vi "Is Complete.vi"(8 "error in (no error)":errorcluster, 11 "Measure Controller in":refnum<class "Measure Controller.lvclass">) -> (0 "error out":errorcluster, 3 "Measure Controller out":refnum<class "Measure Controller.lvclass">)   [LabVIEW 2015, in "Measure Controller.lvclass"]
uses:
  Measure Controller.lvclass
  Measure Controller.lvclass/Measure Controller.ctl
  Measure Object/Measure Object.lvclass/Measure Object.ctl
  Measure Object/Read Counter.vi
  Measure Object/Read Repeat times.vi
  Measure Object/Read Reply to.vi
  Measure Object/Write Counter.vi
  Measure Object Messages/Result Reply Msg/Result Reply Msg.lvclass
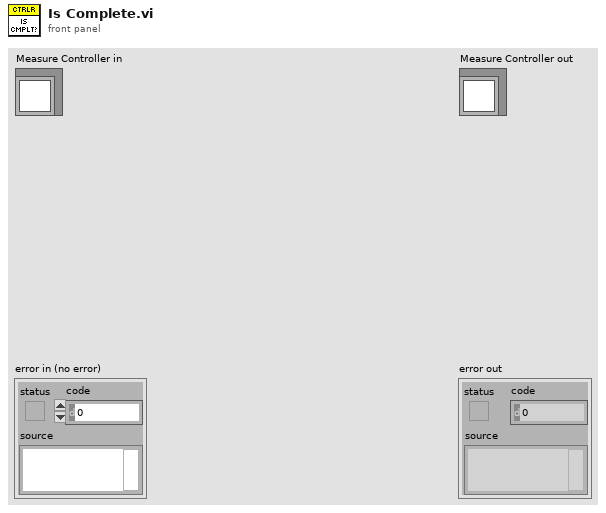
[diagram p1: front panel]
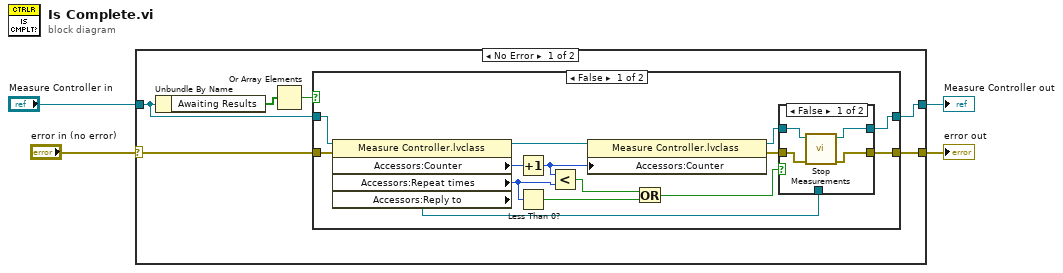
[diagram p0: block diagram]
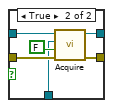
[diagram p2: hidden frame]
diagram:
  n1 = case shown="No Error" "error in (no error)" {
    selector: "error in (no error)" -> [w7 w38]
    tunnel: [w6 w38] -> w3
    tunnel: [w5 w37] -> w1
    tunnel: "Measure Controller in" -> [w8 w37]
    frame No Error {
      n2 = Unbundle By Name(w8) -> ("Awaiting Results"=w10:bool[])
      n3 = Or Array Elements(Boolean array=w10) -> (logical OR=w9:bool)
      n4 = case shown="False" w9 {
        tunnel: w8 -> [w24 w35]
        tunnel: w7 -> [w23 w36]
        tunnel: [w13 w36] -> w6
        tunnel: [w12 w35] -> w5
        frame False {
          n5 = property class="Measure Controller.lvclass"(reference=w24, error in=w23) -> (reference out=w22:refnum<class "Measure Controller.lvclass">, "Accessors:Counter"=w21:i32, "Accessors:Repeat times"=w19:i32, "Accessors:Reply to"=w11:refnum<class "Result Reply Msg.lvclass">)  [unwired: 1 out]
          n6 = Increment(x=w21) -> (x+1=w20:i32)
          n7 = Less Than 0?(x=w19) -> (x < 0?=w17:bool)
          n8 = Less?(x=w20, y=w19) -> (x < y?=w18:bool)
          n9 = property class="Measure Controller.lvclass"(reference=w22, "Accessors:Counter"=w20) -> (reference out=w16:refnum<class "Measure Controller.lvclass">, error out=w15:errorcluster)  [unwired: 1 in]
          n10 = Or(x=w18, y=w17) -> (x .or. y?=w14:bool)
          n11 = case shown="False" w14 {
            tunnel: w16 -> [w25 w34]
            tunnel: w15 -> [w28 w33]
            tunnel: [w27 w32] -> w13
            tunnel: [w26 w31] -> w12
            tunnel: w11 -> [_ w29]
            frame False {
              n12 = call-dynamic "Stop Measurements.vi"("error in (no error)"=w28, "Measure Controller in"=w25) -> ("error out"=w27:errorcluster, "Measure Controller out"=w26:refnum<class "Measure Controller.lvclass">)  [unwired: 8 in]
            }
            frame True {
              n13 = call-dynamic "Acquire.vi"("error in (no error)"=w33, "Initialize"=FALSE, "Reply to"=w29, "Measure Controller in"=w34) -> ("error out"=w32:errorcluster, "Measure Controller out"=w31:refnum<class "Measure Controller.lvclass">)  [unwired: 6 in]
            }
          }
        }
        frame True {
        }
      }
    }
    frame Error {
    }
  }
  "error out" <- w3
  "Measure Controller out" <- w1
